vi "Terminal-PressureSystemLubricateUnit-Setter.vi"(0 "启停":bool=TRUE, 1 "operation timeout (ms)":i32=5000 caption="操作超时（5000毫秒）", 5 "供油流量L":u16, 7 "供油润滑温度T":u16, 11 "error in (no error)":errorcluster caption="错误输入（无错误）") -> (15 "error out":errorcluster caption="错误输出")   [LabVIEW 2014]
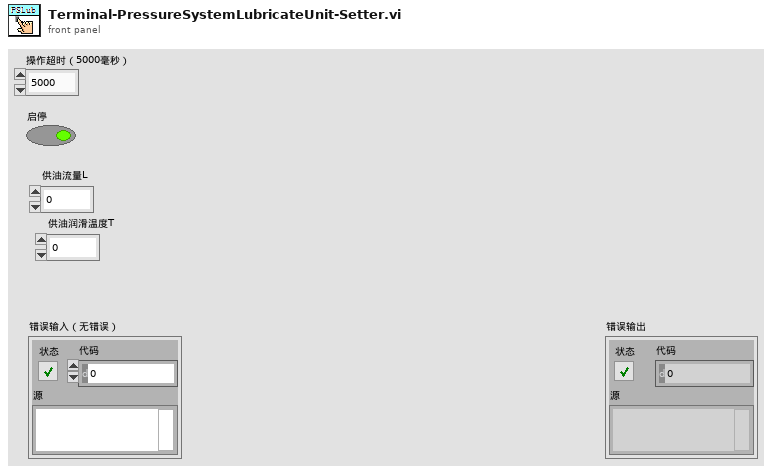
[diagram p1: front panel]
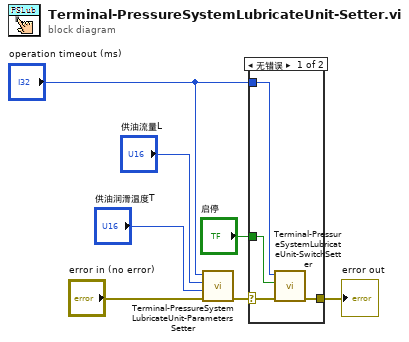
[diagram p0: block diagram]
diagram:
  n1 = call "Terminal-PressureSystemLubricateUnit-ParametersSetter.vi"("error in (no error)"="error in (no error)", "供油润滑温度T"="供油润滑温度T", "供油流量L"="供油流量L", "write operation timeout (ms)"="operation timeout (ms)") -> ("error out"=w6:errorcluster)  [unwired: 7 in]
  n2 = case shown="无错误" w6 {
    selector: w6 -> [w10 w12]
    tunnel: "operation timeout (ms)" -> [w8 _]
    tunnel: [w11 w12] -> w7
    tunnel: "启停" -> [w9 _]
    frame No Error {
      n3 = call "Terminal-PressureSystemLubricateUnit-SwitchSetter.vi"("error in (no error)"=w10, "启停"=w9, "operation timeout (ms)"=w8) -> ("error out"=w11:errorcluster)  [unwired: 8 in]
    }
    frame Error {
    }
  }
  "error out" <- w7
